vi "查询启动项.vi"(8 "error in (no error)":errorcluster caption="错误输入（无错误）", 11 "启动文件路径":path) -> (0 "error out":errorcluster caption="错误输出", 3 "包含启动项":bool)   [LabVIEW 2016]
uses:
  <vilib>/registry/registry.llb/Registry RtKey.ctl
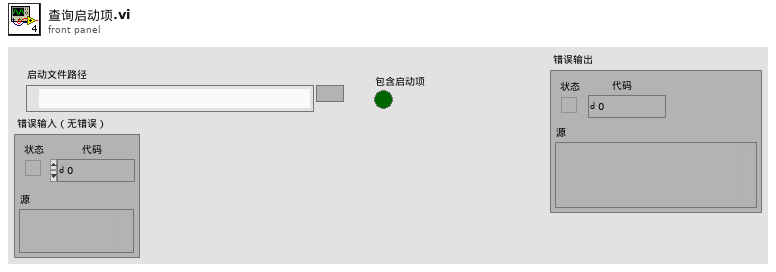
[diagram p1: front panel]
types:
  T1 = typedef "Registry RtKey.ctl" = enum32{"HKEY_CLASSES_ROOT", "HKEY_CURRENT_USER", "HKEY_LOCAL_MACHINE", "HKEY_USERS", "HKEY_PERFORMANCE_DATA", "HKEY_CURRENT_CONFIG", "HKEY_DYN_DATA"}
  T2 = typedef "Registry refnum.ctl" = refnum<k1>
  T3 = cluster{"numValues":i32, "maxValueNameLen":i32, "maxValueDataLen":i32}
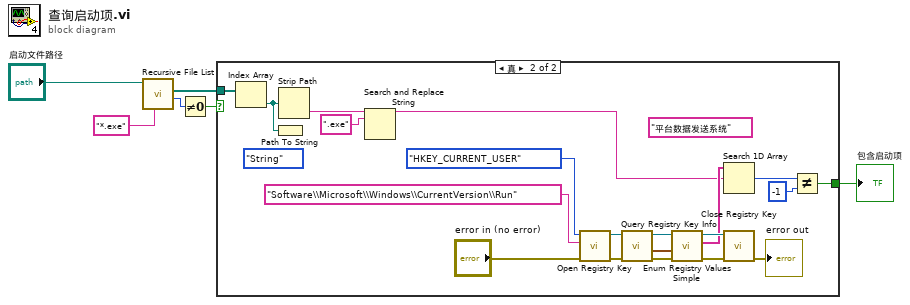
[diagram p0: block diagram]
diagram:
  n1 = call <vilib>:"Recursive File List.vi"("pattern"="*.exe", "Folder Path"="启动文件路径") -> ("Number of Files"=w4:i32, "All Files in Dir"=w5:path[])  [unwired: 5 in, 3 out]
  n2 = Not Equal To 0?(x=w4) -> (x != 0?=w3:bool)
  n3 = case shown="真" w3 {
    tunnel: w5 -> [_ w26]
    tunnel: [_ w10] -> w2
    frame False {
    }
    frame True {
      (unwired) "平台数据发送系统"
      (unwired) enum16{"String", "Binary", "DWORD"}."String" ("simple data type")
      n4 = Index Array(array=w26) -> (element=w25:path)  [unwired: 1 in]
      n5 = Path To String(path=w25) -> ()  [unwired: 1 out]
      n6 = Strip Path(path=w25) -> (name=w24:string)  [unwired: 1 out]
      n7 = Search and Replace String(input string=w24, search string=".exe" ("搜索字符串")) -> (result string=w7:string)  [unwired: 6 in, 3 out]
      n8 = call <vilib>:"Open Registry Key.vi"("error in (no error)"="error in (no error)", "subkey"="Software\\Microsoft\\Windows\\CurrentVersion\\Run", "root key (HKEY_LOCAL_MACHINE)"=Registry_RtKey."HKEY_CURRENT_USER") -> ("error out"=w19:errorcluster, "refnum out"=w20:T2)  [unwired: 7 in]
      n9 = call <vilib>:"Query Registry Key Info.vi"("error in (no error)"=w19, "refnum"=w20) -> ("error out"=w16:errorcluster, "value info"=w17:T3, "refnum out"=w18:T2)  [unwired: 5 in, 2 out]
      n10 = call <vilib>:"Enum Registry Values Simple.vi"("error in (no error)"=w16, "value info"=w17, "refnum"=w18) -> ("error out"=w14:errorcluster, "values"=w13:string[], "refnum out"=w15:T2)  [unwired: 3 in, 3 out]
      n11 = Search 1D Array(1D array=w13, element=w7) -> (index of element=w12:i32)  [unwired: 1 in]
      n12 = call <vilib>:"Close Registry Key.vi"("error in (no error)"=w14, "refnum"=w15) -> ("error out"=→"error out":errorcluster)  [unwired: 5 in]
      n13 = Not Equal?(x=w12, y=-1) -> (x != y?=w10:bool)
    }
  }
  "包含启动项" <- w2
